vi "SA40144D.20210720 vacuum 1D only.vi"() -> ()   [LabVIEW 2020]
uses:
  <vilib>/Analysis/baseanly.llb/Mean (DBL).vi
  <userlib>/_OpenG.lib/file/file.llb/Build Path - Traditional__ogtk.vi
  <userlib>/LevyLab/LV to ITX/Data/Data.lvclass
  <userlib>/LevyLab/XY Utilities/xy_utilities.lvlib
  <vilib>/Analysis/NI_AALBase.lvlib
panel:
  in  "Tab Control":enum32{"Page 1", "Page 2"}(tab)
  out "G4T vs t  - R Channel":T1(graph)
  out "G2T vs t - R channel":T1(graph)
  out "G2T vs t - X channel":T1(graph)
  out "G4T vs t - X channel":T1(graph)
  out "Temp vs t":T1(graph)
  out "Arrhenius":T1(graph)
  out "R6 - dV":T1(graph)
  out "R5 - I-":T1(graph)
  out "Y6 - dV":T1(graph)
  out "Y5 - I-":T1(graph)
  out "X5 - I-":T1(graph)
  out "X6 - dV":T1(graph)
  in  "Temps to keep (Lifespan)":i32=26
  out "E_a":dbl[](array[numeric])
  in  "Temps to keep (Arrhenius fit)":i32=26
  in  "Source Voltage":dbl=0.1
  in  "Init Temp":i32=275
  in  "Temp Step":i32=5
  in  "Final Temp":i32=400
  in  "Data File":path=path "G:/My Drive/ansom/Data/PPMS 2/SA40144D.20210720/00 - test/SA40144D.20210720.275K.dat"
  in  "Trimming":i32=400
  in  "Update":bool
  in  "OK":bool
  out "error out":errorcluster
  in  "error in (no error)":errorcluster
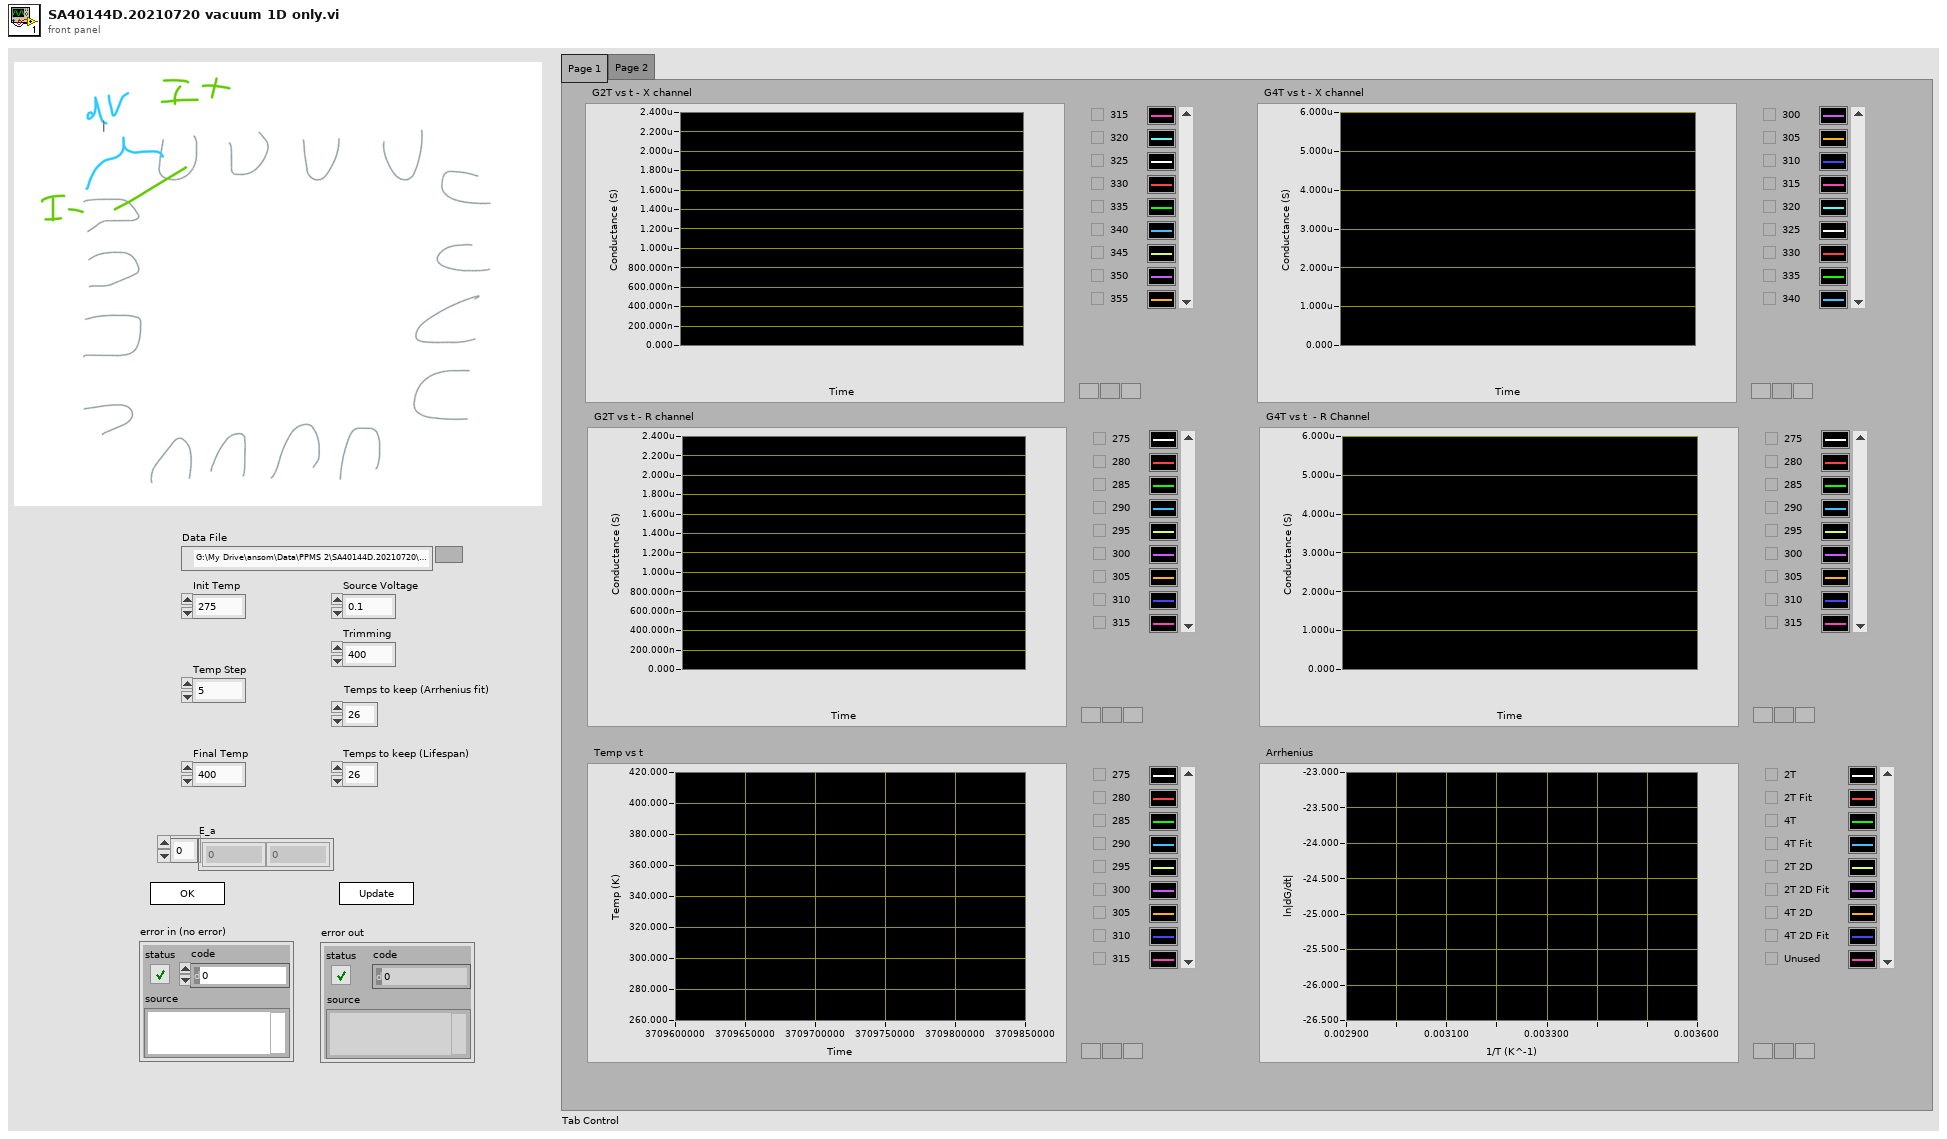
[diagram p1: front panel]
types:
  T1 = cluster{"Data":dbl[], "Best Exponential Fit":dbl[]}[]
  T2 = enum32{"Invalid", "Standard", "Closed", "Hidden", "Minimized", "Maximized"}
  T3 = enum32{"invalid app kind", "Development System", "Run Time System", "Student Edition", "Embedded LabVIEW", "Evaluation", "Custom"}
  T4 = cluster{"Core":cluster{"Current VI Reference":refnum<vi>, "Close Panel on Exit?":bool}, "G2T 1D":cluster{dbl[], dbl[]}[], "G4T 1D":cluster{dbl[], dbl[]}[], "X11":cluster{dbl[], dbl[]}[], "X15":cluster{dbl[], dbl[]}[], "Temp":cluster{dbl[], dbl[]}[], "G2T BG":cluster{dbl[], dbl[]}[], "Source Voltage":dbl, "Final Temp":i32, "Init Temp":i32, "Temp Step":i32, "Data File":path, "Trimming":i32}
  T5 = cluster{"Current VI Reference":refnum<vi>, "Close Panel on Exit?":bool}
  T6 = typedef "Data.lvclass/Dictionary--cluster.ctl" = cluster{"key":string, "value":variant}
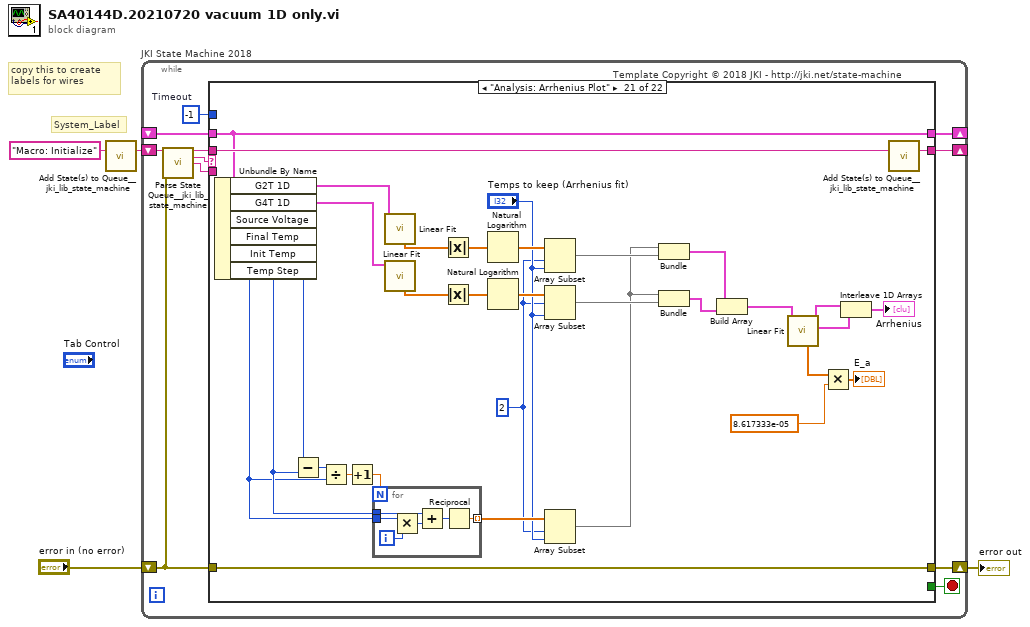
[diagram p0: block diagram]
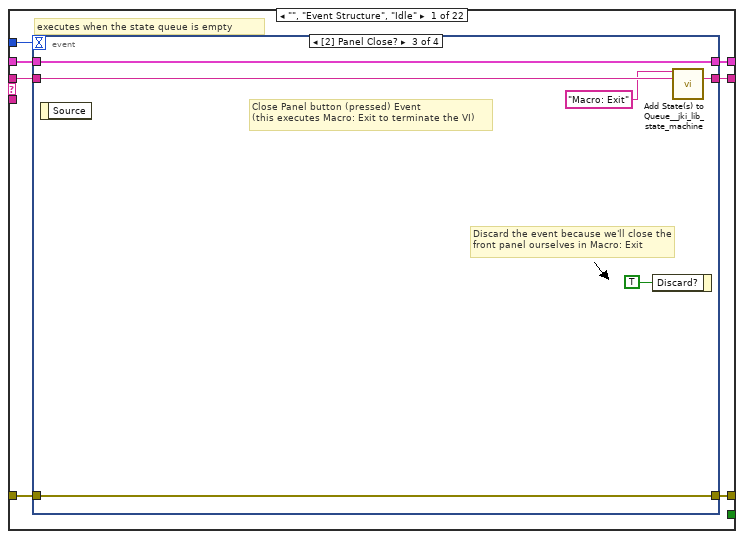
[diagram p2: hidden frame]
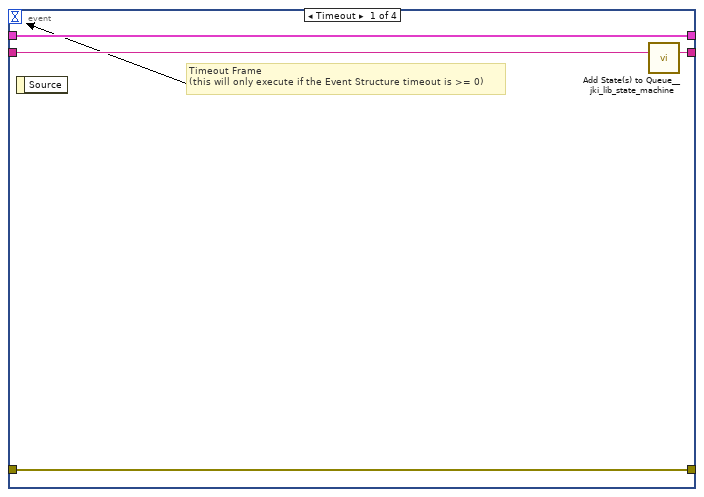
[diagram p3: hidden frame]
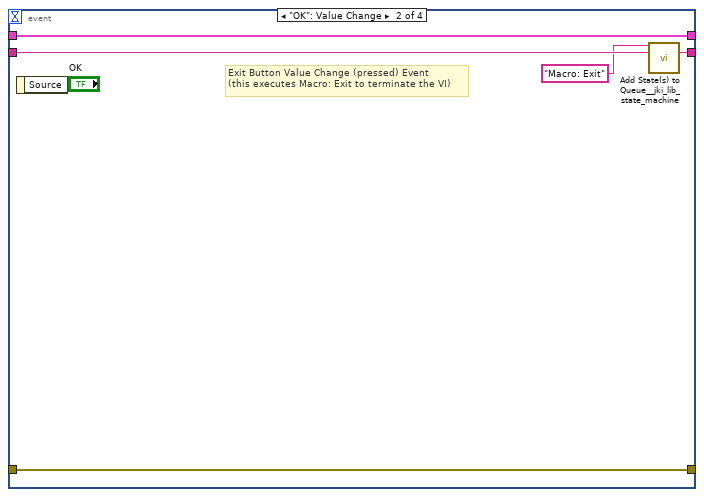
[diagram p4: hidden frame]
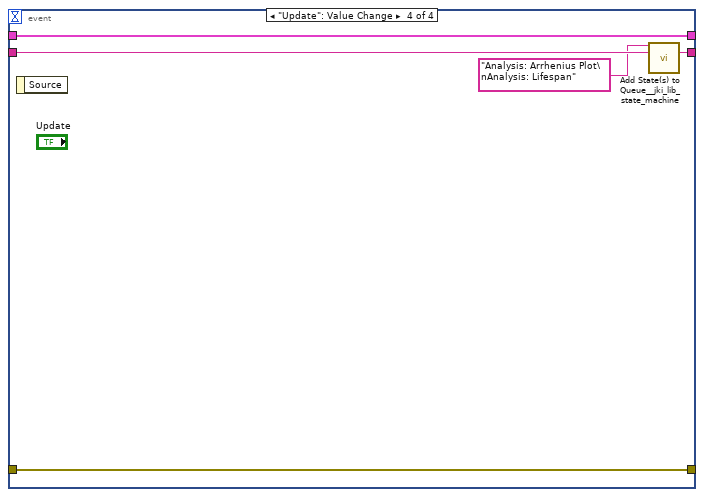
[diagram p5: hidden frame]
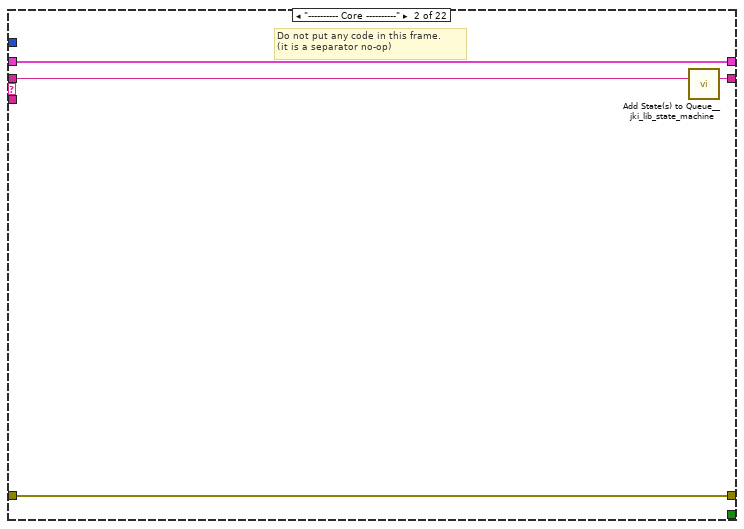
[diagram p6: hidden frame]
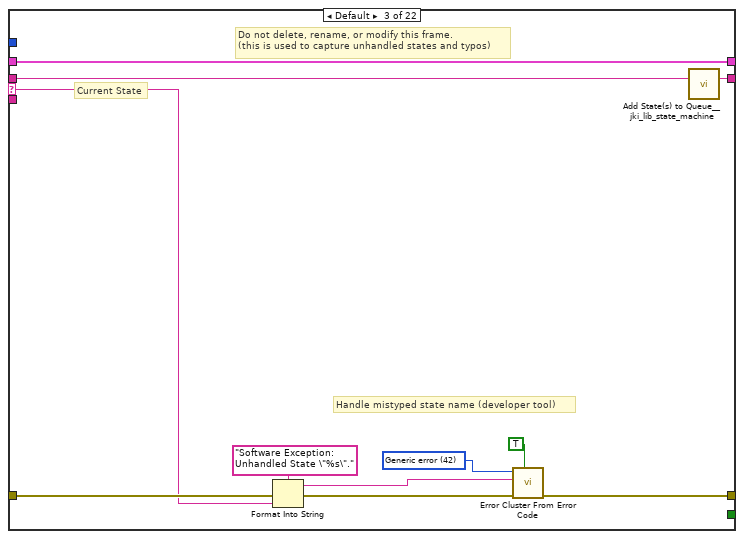
[diagram p7: hidden frame]
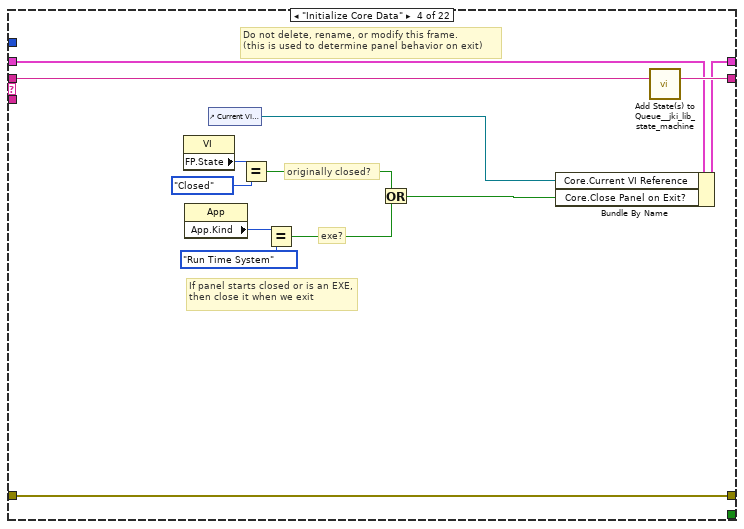
[diagram p8: hidden frame]
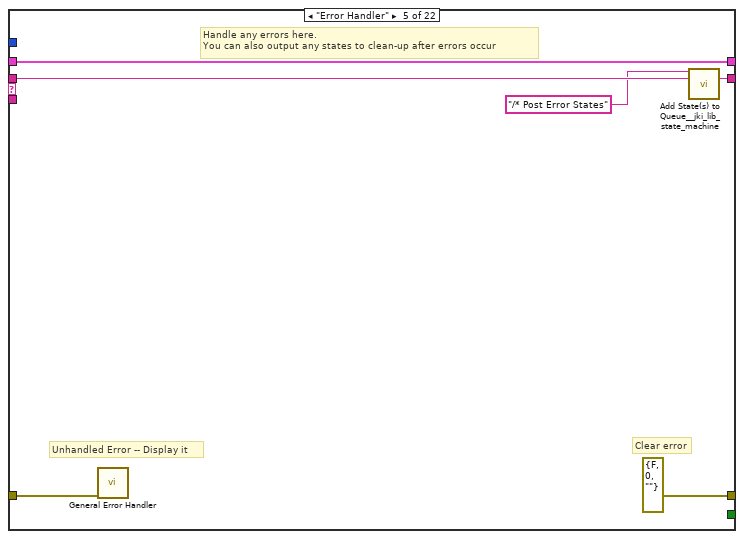
[diagram p9: hidden frame]
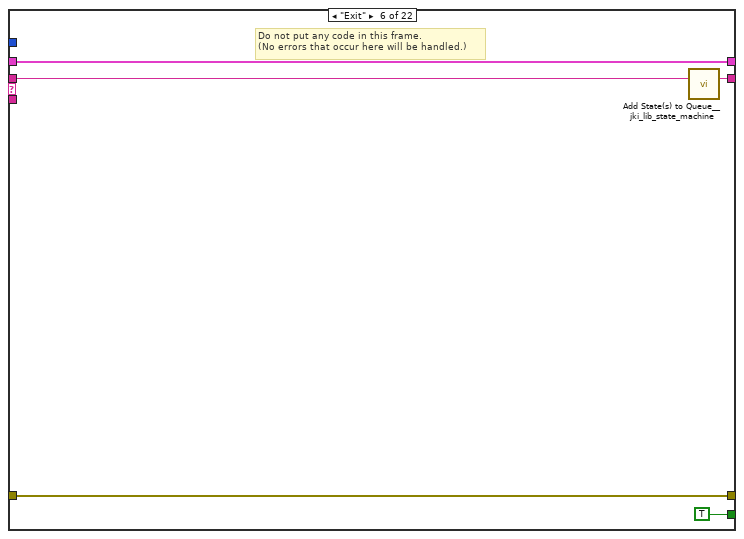
[diagram p10: hidden frame]
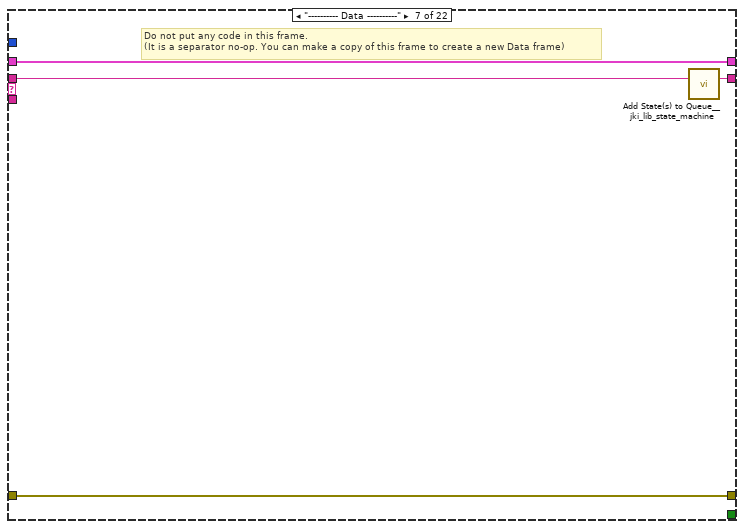
[diagram p11: hidden frame]
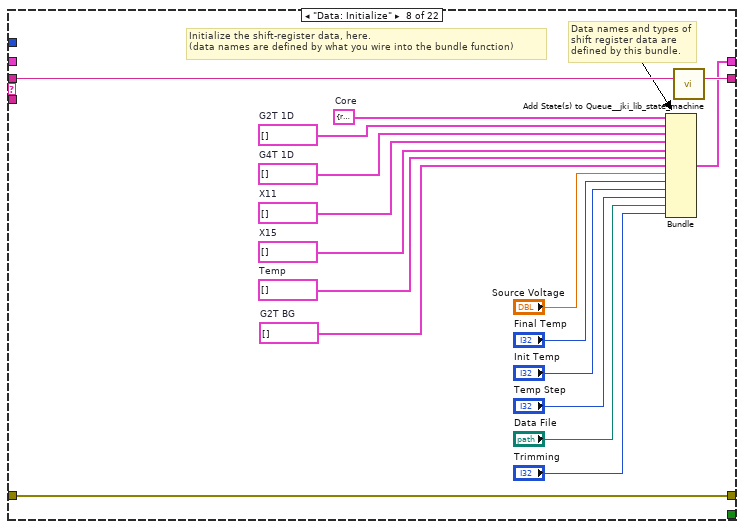
[diagram p12: hidden frame]
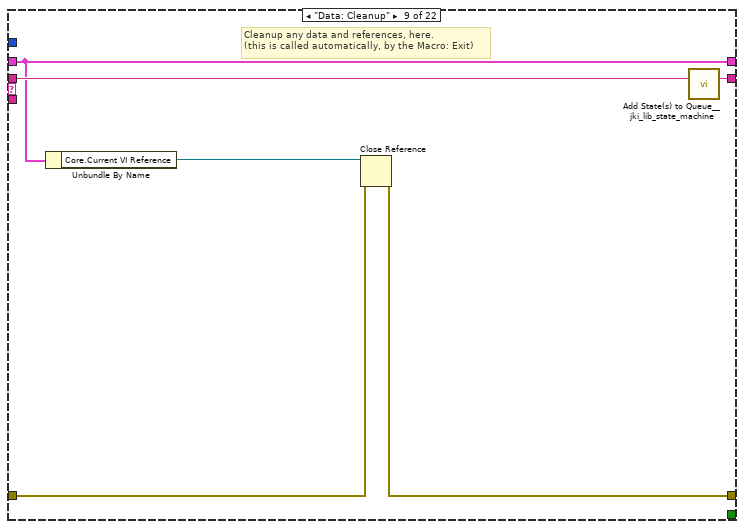
[diagram p13: hidden frame]
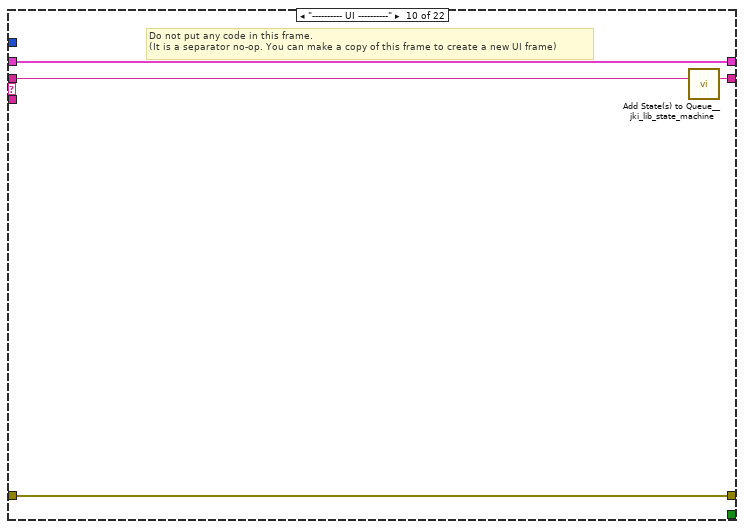
[diagram p14: hidden frame]
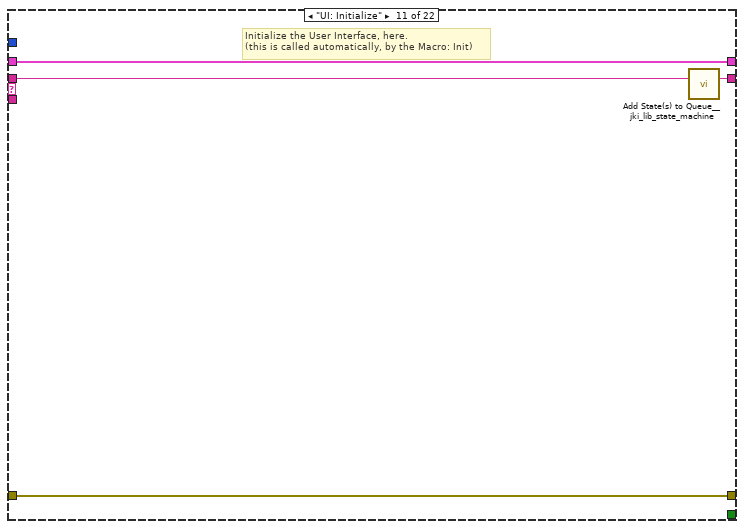
[diagram p15: hidden frame]
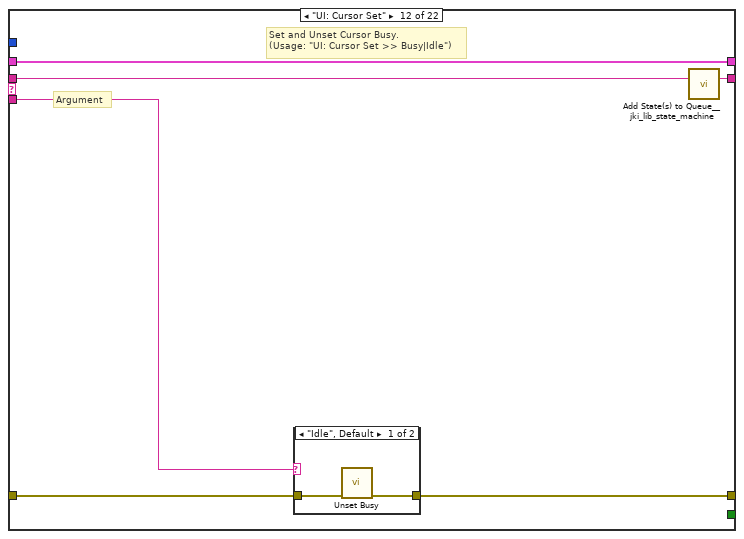
[diagram p16: hidden frame]
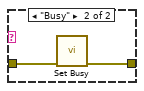
[diagram p17: hidden frame]
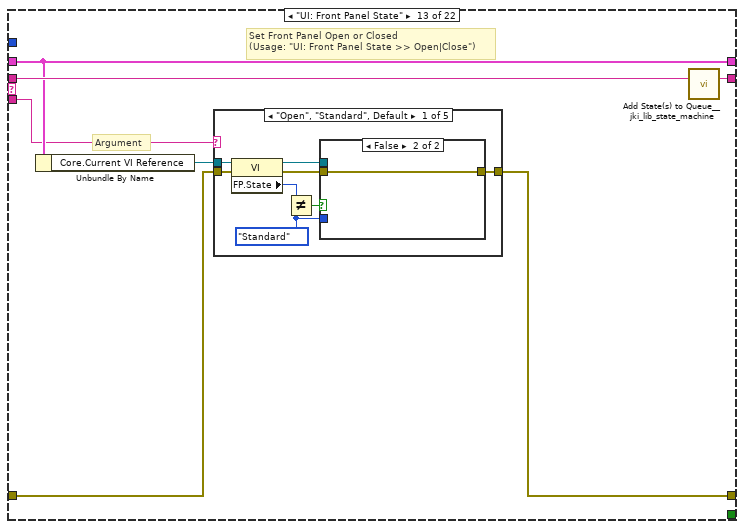
[diagram p18: hidden frame]
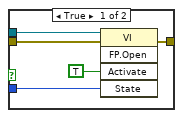
[diagram p19: hidden frame]
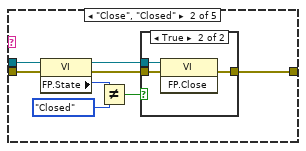
[diagram p20: hidden frame]
diagram:
  # "copy this to create labels for wires"
  # "System_Label"
  n1 = call <vilib>:"Add State(s) to Queue__jki_lib_state_machine.vi"("State(s) in (\"\")"="Macro: Initialize") -> ("States Out"=w4:string)  [unwired: 14 in]
  n2 = while "JKI State Machine 2018" {
    shift-right: [w8] -> _
    shift-left: _ -> [w7]
    shift-right: [w11] -> w1
    shift-left: "error in (no error)" -> [w5]
    shift-right: [w10] -> _
    shift-left: w4 -> [w12]
    stop <- w9 stop-if-true
    w6 = -1  # Timeout
    # "Template Copyright © 2018 JKI - http://jki.net/state-machine"
    n3 = call <vilib>:"Parse State Queue__jki_lib_state_machine.vi"("State Queue"=w12, "Error In (no error)"=w5) -> ("Remaining States"=w14:string, "Current State"=w15:string, "Arguments"=w13:string)  [unwired: 11 in]
    n4 = case shown="\"Analysis: Arrhenius Plot\"" w15 {
      selector: w15 -> [_ _ w47 _ _ _ _ _ _ _ _ _ _ _ _ _ _ _ _ _ _ _]
      tunnel: w14 -> [w22 w46 w51 w70 w76 w81 w85 w102 w108 w112 w116 w122 w133 w202 w207 w217 w221 w242 w315 w359 w392 w430]
      tunnel: w13 -> [_ _ _ _ _ _ _ _ _ _ _ w117 w127 _ _ _ _ _ _ _ _ _]
      tunnel: w7 -> [w20 w43 w49 w63 w73 w79 w82 _ w103 w109 w114 w120 w129 w199 w204 w214 w218 w236 w309 w356 w389 w416]
      tunnel: [w19 w44 w53 w67 errorcluster {"status"=FALSE, "code"=0, "source"=""} ("error out") w78 w83 w99 w104 w110 w113 w118 w130 w200 w205 w215 w219 w238 w311 w357 w390 w428] -> w11
      tunnel: w5 -> [w18 w44 w52 w67 w72 w78 w83 w99 w105 w110 w113 w119 w131 w200 w205 w215 w219 w238 w311 w357 w390 w428]
      tunnel: [w21 w45 w50 w69 w75 w80 w84 w101 w107 w111 w115 w121 w132 w201 w206 w216 w220 w241 w314 w358 w391 w429] -> w10
      tunnel: [_ _ _ _ _ TRUE _ _ _ _ _ _ _ _ _ _ _ _ _ _ _ _] -> w9
      tunnel: [w17 w43 w49 w68 w73 w79 w82 w100 w103 w109 w114 w120 w129 w199 w204 w214 w218 w237 w310 w356 w389 w416] -> w8
      tunnel: w6 -> [w16 _ _ _ _ _ _ _ _ _ _ _ _ _ _ _ _ _ _ _ _ _]
      frame "", "Event Structure", "Idle" {
        # "executes when the state queue is empty"
        n5 = event shown="[2] Panel Close?" {
          selector: _ -> [_ _ _ _]
          dyn-events: _ -> [_ _ _ _]
          timeout: w16 -> [_ _ _ _]
          tunnel: w22 -> [w26 w31 w37 w41]
          tunnel: [w25 w30 w36 w40] -> w21
          tunnel: w20 -> [w23 w28 w34 w42]
          tunnel: [w24 w29 w35 w38] -> w19
          tunnel: w18 -> [w24 w29 w35 w38]
          tunnel: [w23 w28 w34 w42] -> w17
          event Timeout {
            # "Timeout Frame\n(this will only execute if the Event Structure timeout is >= 0)"
            n6 = event-data() -> ()  [unwired: 1 in, 1 out]
            n7 = call <vilib>:"Add State(s) to Queue__jki_lib_state_machine.vi"("State(s) in (\"\")"=w26) -> ("States Out"=w25:string)  [unwired: 14 in]
          }
          event "OK": Value Change {
            # "Exit Button Value Change (pressed) Event\n(this executes Macro: Exit to terminate the VI)"
            n8 = event-data() -> ()  [unwired: 1 in, 1 out]
            n9 = call <vilib>:"Add State(s) to Queue__jki_lib_state_machine.vi"("State(s) in Front (\"\")"="Macro: Exit", "State(s) in (\"\")"=w31) -> ("States Out"=w30:string)  [unwired: 13 in]
          }
          event Panel Close? {
            # "Discard the event because we'll close the front panel ourselves in Macro: Exit"
            # "Close Panel button (pressed) Event\n(this executes Macro: Exit to terminate the VI)"
            n10 = event-data() -> ()  [unwired: 1 in, 1 out]
            n11 = event-data("Discard?"=TRUE) -> ()  [unwired: 1 in, 1 out]
            n12 = call <vilib>:"Add State(s) to Queue__jki_lib_state_machine.vi"("State(s) in Front (\"\")"="Macro: Exit", "State(s) in (\"\")"=w37) -> ("States Out"=w36:string)  [unwired: 13 in]
          }
          event "Update": Value Change {
            n13 = event-data() -> ()  [unwired: 1 in, 1 out]
            n14 = call <vilib>:"Add State(s) to Queue__jki_lib_state_machine.vi"("State(s) in Front (\"\")"="Analysis: Arrhenius Plot\nAnalysis: Lifespan" ("State(s) in Front (\"\")"), "State(s) in (\"\")"=w41) -> ("States Out"=w40:string)  [unwired: 13 in]
          }
        }
      }
      frame "---------- Core ----------" {
        # "Do not put any code in this frame.\n(it is a separator no-op)"
        n15 = call <vilib>:"Add State(s) to Queue__jki_lib_state_machine.vi"("State(s) in (\"\")"=w46) -> ("States Out"=w45:string)  [unwired: 14 in]
      }
      frame Default {
        w56 = 42 items=["No error", "Argument error", "Memory is full", "Out of zone", "End of file", "File already open", "Generic file I/O error", "File not found", "File permission error", "Disk is full", "Duplicate path", "Too many files open", "System feature not enabled", "Resource file not found", "Cannot add resource", "Resource not found", "Image not found", "Image memory error", "Pen does not exist", "Config type invalid", "Config token not found", "Config parse error", "Config memory error", "Bad external code format", "Bad external code offset", "External code not present", "Null window", "Destroy window error", "Null menu", "Print aborted", "Bad print record", "Print driver error", "Windows error during printing", "Memory error during printing", "Print dialog error", "Generic print error", "Invalid device refnum", "Device not found", "Device parameter error", "Device unit error", "Cannot open device", "Device call aborted", "Generic error", "Cancelled by user", "Object ID too low", "Object ID too high", "Object not in heap", "Unknown heap", "Unknown object (invalid DefProc)", "Unknown object (DefProc not in table)", "Message out of range", "Invalid (null) method", "Unknown message", "Manager call not supported", "Bad address", "Network operation in progress", "Network operation timed out", "Connection is busy", "Network attribute not supported", "Network error", "Address in use", "System out of memory", "Connection aborted", "Connection refused", "Not connected", "Already connected", "Connection closed", "Initialization error (interapplication manager)", "Bad occurrence", "Wait on unbound occurrence handler", "Occurrence queue overflow", "Datalog type conflict", "Unused", "Unrecognized type (interapplication manager)", "Memory corrupt", "Failed to make temporary DLL", "Old CIN version", "Drag socket not found", "Failed to load drop-object", "Failed to register OLE object", "Failed to release OLE object", "Format specifier type mismatch", "Unknown format specifier", "Too few format specifiers", "Too many format specifiers", "Scan failed", "Newer CIN version", "Error converting to variant", "Runtime menu error", "Password tampered", "Variant attribute not found", "Incompatible variant data type", "Event data is not available", "Event Store is not present", "Occurrence is not found", "Event Queue is not created", "Event info is not available", "Refnum passed is NULL", "Error retrieving Class GUID", "Error retrieving CoClass GUID", "Error retrieving TypeLib GUID.", "Bad built application magic bytes.", "Specific driver is different from the specific driver associated with the Logical Name.", "There is no session opened to the class driver.", "Max Error", "MAX - Error with config objects", "MAX - Error loading configuration", "MAX - Group not supported"]
        # "Current State"
        # "Do not delete, rename, or modify this frame.\n(this is used to capture unhandled states and typos)"
        # "Handle mistyped state name (developer tool)"
        n16 = Format Into String(format string="Software Exception: Unhandled State \"%s\"." ("message"), error in=w52, w47) -> (resulting string=w55:string, error out=w54:errorcluster)  [unwired: 1 in]
        n17 = call <vilib>:"Error Cluster From Error Code.vi"("show call chain? (False)"=TRUE, "error in (no error)"=w54, "error message (\"\")"=w55, "error code (0)"=w56) -> ("error out"=w53:errorcluster)  [unwired: 5 in]
        n18 = call <vilib>:"Add State(s) to Queue__jki_lib_state_machine.vi"("State(s) in (\"\")"=w51) -> ("States Out"=w50:string)  [unwired: 14 in]
      }
      frame "Initialize Core Data" {
        # "Do not delete, rename, or modify this frame.\n(this is used to determine panel behavior on exit)"
        # "originally closed?"
        # "exe?"
        # "If panel starts closed or is an EXE, then close it when we exit"
        n19 = property class="VI"() -> ("FP.State"=w60:T2)  [unwired: 2 in, 2 out]
        n20 = property class="App"() -> ("App.Kind"=w66:T3)  [unwired: 2 in, 2 out]
        n21 = control-ref of="Current VI Reference"() -> (w61:refnum<vi>)
        n22 = Equal?(x=w60, y=T2."Closed" ("Front Panel Window:State")) -> (x = y?=w58:bool)
        n23 = Equal?(x=w66, y=T3."Run Time System" ("Application:Kind")) -> (x = y?=w64:bool)
        n24 = Or(x=w58, y=w64) -> (x .or. y?=w62:bool)
        n25 = Bundle By Name(cluster=w63, "Core.Current VI Reference"=w61, "Core.Close Panel on Exit?"=w62) -> (w68:T4)
        n26 = call <vilib>:"Add State(s) to Queue__jki_lib_state_machine.vi"("State(s) in (\"\")"=w70) -> ("States Out"=w69:string)  [unwired: 14 in]
      }
      frame "Error Handler" {
        # "Unhandled Error -- Display it"
        # "Handle any errors here.\nYou can also output any states to clean-up after errors occur"
        # "Clear error"
        n27 = call <vilib>:"General Error Handler.vi"("error in (no error)"=w72) -> ()  [unwired: 10 in, 5 out]
        n28 = call <vilib>:"Add State(s) to Queue__jki_lib_state_machine.vi"("State(s) in Front (\"\")"="/* Post Error States", "State(s) in (\"\")"=w76) -> ("States Out"=w75:string)  [unwired: 13 in]
      }
      frame "Exit" {
        # "Do not put any code in this frame.\n(No errors that occur here will be handled.)"
        n29 = call <vilib>:"Add State(s) to Queue__jki_lib_state_machine.vi"("State(s) in (\"\")"=w81) -> ("States Out"=w80:string)  [unwired: 14 in]
      }
      frame "---------- Data ----------" {
        # "Do not put any code in this frame.\n(It is a separator no-op. You can make a copy of this frame to create a new Data frame)"
        n30 = call <vilib>:"Add State(s) to Queue__jki_lib_state_machine.vi"("State(s) in (\"\")"=w85) -> ("States Out"=w84:string)  [unwired: 14 in]
      }
      frame "Data: Initialize" {
        w86 = cluster{dbl[], dbl[]}[] []  # G2T BG
        w87 = cluster{dbl[], dbl[]}[] []  # Temp
        w96 = cluster{dbl[], dbl[]}[] []  # X15
        w95 = cluster{dbl[], dbl[]}[] []  # X11
        w94 = cluster{dbl[], dbl[]}[] []  # G4T 1D
        w93 = cluster{dbl[], dbl[]}[] []  # G2T 1D
        w98 = T5 {"Current VI Reference"=refnum, "Close Panel on Exit?"=FALSE}  # Core
        # "Data names and types of shift register data are defined by this bundle."
        # "Initialize the shift-register data, here.\n(data names are defined by what you wire into the bundle function)"
        n31 = Bundle("Core"=w98, "G2T 1D"=w93, "G4T 1D"=w94, "X11"=w95, "X15"=w96, "Temp"=w87, "G2T BG"=w86, "Source Voltage"="Source Voltage", "Final Temp"="Final Temp", "Init Temp"="Init Temp", "Temp Step"="Temp Step", "Data File"="Data File", "Trimming"="Trimming") -> (w100:T4)  [unwired: 1 in]
        n32 = call <vilib>:"Add State(s) to Queue__jki_lib_state_machine.vi"("State(s) in (\"\")"=w102) -> ("States Out"=w101:string)  [unwired: 14 in]
      }
      frame "Data: Cleanup" {
        # "Cleanup any data and references, here.\n(this is called automatically, by the Macro: Exit)"
        n33 = Unbundle By Name(w103) -> ("Core.Current VI Reference"=w106:refnum<vi>)
        n34 = Close Reference(reference=w106, error in (no error)=w105) -> (error out=w104:errorcluster)
        n35 = call <vilib>:"Add State(s) to Queue__jki_lib_state_machine.vi"("State(s) in (\"\")"=w108) -> ("States Out"=w107:string)  [unwired: 14 in]
      }
      frame "---------- UI ----------" {
        # "Do not put any code in this frame.\n(It is a separator no-op. You can make a copy of this frame to create a new UI frame)"
        n36 = call <vilib>:"Add State(s) to Queue__jki_lib_state_machine.vi"("State(s) in (\"\")"=w112) -> ("States Out"=w111:string)  [unwired: 14 in]
      }
      frame "UI: Initialize" {
        # "Initialize the User Interface, here.\n(this is called automatically, by the Macro: Init)"
        n37 = call <vilib>:"Add State(s) to Queue__jki_lib_state_machine.vi"("State(s) in (\"\")"=w116) -> ("States Out"=w115:string)  [unwired: 14 in]
      }
      frame "UI: Cursor Set" {
        # "Argument"
        # "Set and Unset Cursor Busy.\n(Usage: \"UI: Cursor Set >> Busy|Idle\")"
        n38 = case shown="\"Idle\", Default" w117 {
          tunnel: w119 -> [w124 w126]
          tunnel: [w123 w125] -> w118
          frame "Idle", Default {
            n39 = call <vilib>:"Unset Busy.vi"("error in (no error)"=w124) -> ("error out"=w123:errorcluster)  [unwired: 10 in]
          }
          frame "Busy" {
            n40 = call <vilib>:"Set Busy.vi"("error in (no error)"=w126) -> ("error out"=w125:errorcluster)  [unwired: 9 in, 1 out]
          }
        }
        n41 = call <vilib>:"Add State(s) to Queue__jki_lib_state_machine.vi"("State(s) in (\"\")"=w122) -> ("States Out"=w121:string)  [unwired: 14 in]
      }
      frame "UI: Front Panel State" {
        # "Argument"
        # "Set Front Panel Open or Closed\n(Usage: \"UI: Front Panel State >> Open|Close\")"
        n42 = Unbundle By Name(w129) -> ("Core.Current VI Reference"=w128:refnum<vi>)
        n43 = case shown="\"Open\", \"Standard\", Default" w127 {
          tunnel: w131 -> [w139 w154 w165 w178 w191]
          tunnel: [w141 w155 w167 w180 w193] -> w130
          tunnel: w128 -> [w140 w152 w166 w179 w192]
          frame "Open", "Standard", Default {
            w134 = T2."Standard" ("State")
            n44 = property class="VI"(reference=w140, error in=w139) -> (reference out=w137:refnum<vi>, error out=w138:errorcluster, "FP.State"=w136:T2)
            n45 = Not Equal?(x=w136, y=w134) -> (x != y?=w135:bool)
            n46 = case shown="False" w135 {
              tunnel: [w145 w147] -> w141
              tunnel: w138 -> [w144 w147]
              tunnel: w137 -> [w143 _]
              tunnel: w134 -> [w142 _]
              frame True {
                n47 = invoke class="VI" method="FP.Open"(reference=w143, error in=w144, "Activate"=TRUE, "State"=w142) -> (error out=w145:errorcluster)  [unwired: 1 in, 4 out]
              }
              frame False {
              }
            }
          }
          frame "Close", "Closed" {
            n48 = property class="VI"(reference=w152, error in=w154) -> (reference out=w151:refnum<vi>, error out=w153:errorcluster, "FP.State"=w149:T2)
            n49 = Not Equal?(x=w149, y=T2."Closed" ("Front Panel Window:State")) -> (x != y?=w148:bool)
            n50 = case shown="True" w148 {
              tunnel: [w156 w159] -> w155
              tunnel: w153 -> [w156 w158]
              tunnel: w151 -> [_ w157]
              frame False {
              }
              frame True {
                n51 = invoke class="VI" method="FP.Close"(reference=w157, error in=w158) -> (error out=w159:errorcluster)  [unwired: 1 in, 2 out]
              }
            }
          }
          frame "Hidden", "Hide" {
            w160 = T2."Hidden" ("State")
            n52 = property class="VI"(reference=w166, error in=w165) -> (reference out=w163:refnum<vi>, error out=w164:errorcluster, "FP.State"=w162:T2)
            n53 = Not Equal?(x=w162, y=w160) -> (x != y?=w161:bool)
            n54 = case shown="True" w161 {
              tunnel: [w171 w172] -> w167
              tunnel: w164 -> [w170 w172]
              tunnel: w163 -> [w169 _]
              tunnel: w160 -> [w168 _]
              frame True {
                n55 = invoke class="VI" method="FP.Open"(reference=w169, error in=w170, "State"=w168) -> (error out=w171:errorcluster)  [unwired: 2 in, 4 out]
              }
              frame False {
              }
            }
          }
          frame "Minimize", "Minimized" {
            w173 = T2."Minimized" ("State")
            n56 = property class="VI"(reference=w179, error in=w178) -> (reference out=w176:refnum<vi>, error out=w177:errorcluster, "FP.State"=w175:T2)
            n57 = Not Equal?(x=w175, y=w173) -> (x != y?=w174:bool)
            n58 = case shown="True" w174 {
              tunnel: [w184 w185] -> w180
              tunnel: w177 -> [w183 w185]
              tunnel: w176 -> [w182 _]
              tunnel: w173 -> [w181 _]
              frame True {
                n59 = invoke class="VI" method="FP.Open"(reference=w182, error in=w183, "State"=w181) -> (error out=w184:errorcluster)  [unwired: 2 in, 4 out]
              }
              frame False {
              }
            }
          }
          frame "Maximize", "Maximized" {
            w186 = T2."Maximized" ("State")
            n60 = property class="VI"(reference=w192, error in=w191) -> (reference out=w189:refnum<vi>, error out=w190:errorcluster, "FP.State"=w188:T2)
            n61 = Not Equal?(x=w188, y=w186) -> (x != y?=w187:bool)
            n62 = case shown="True" w187 {
              tunnel: [w197 w198] -> w193
              tunnel: w190 -> [w196 w198]
              tunnel: w189 -> [w195 _]
              tunnel: w186 -> [w194 _]
              frame True {
                n63 = invoke class="VI" method="FP.Open"(reference=w195, error in=w196, "State"=w194) -> (error out=w197:errorcluster)  [unwired: 2 in, 4 out]
              }
              frame False {
              }
            }
          }
        }
        n64 = call <vilib>:"Add State(s) to Queue__jki_lib_state_machine.vi"("State(s) in (\"\")"=w133) -> ("States Out"=w132:string)  [unwired: 14 in]
      }
      frame "---------- Macro ----------" {
        # "Do not put any code in this frame.\n(It is a separator no-op. You can make a copy of this frame to create a new Macro frame)"
        n65 = call <vilib>:"Add State(s) to Queue__jki_lib_state_machine.vi"("State(s) in (\"\")"=w202) -> ("States Out"=w201:string)  [unwired: 14 in]
      }
      frame "Macro: Initialize" {
        # "Initialization Macro\n(This is called once, when the VI starts)"
        n66 = call <vilib>:"Add State(s) to Queue__jki_lib_state_machine.vi"("State(s) in Front (\"\")"="Data: Initialize\nInitialize Core Data\nUI: Initialize\nUI: Front Panel State >> Open\nAnalysis: Load 1D\nAnalysis: Load X\nAnalysis: Plot G vs t\nAnalysis: Arrhenius Plot\nAnalysis: Lifespan", "State(s) in (\"\")"=w207) -> ("States Out"=w206:string)  [unwired: 13 in]
      }
      frame "Macro: Exit" {
        # "Exit Macro\n(This is called once, when the VI exits)"
        n67 = Unbundle By Name(w214) -> ("Core.Close Panel on Exit?"=w213:bool)
        n68 = Select(t="UI: Front Panel State >> Close", s=w213, f="") -> (s? t:f=w210:string)
        n69 = call <vilib>:"Add State(s) to Queue__jki_lib_state_machine.vi"("State(s) in (\"\")"=w210, "State(s) at Back (\"\")"="Data: Cleanup\nExit") -> ("States Out"=w208:string)  [unwired: 13 in]
        n70 = call <vilib>:"Add State(s) to Queue__jki_lib_state_machine.vi"("State(s) in Front (\"\")"=w208, "State(s) in (\"\")"=w217) -> ("States Out"=w216:string)  [unwired: 13 in]
      }
      frame "---------- Analysis ----------" {
        # "Template Separator\n(You can make a copy of, or modify, this frame)"
        n71 = call <vilib>:"Add State(s) to Queue__jki_lib_state_machine.vi"("State(s) in (\"\")"=w221) -> ("States Out"=w220:string)  [unwired: 14 in]
      }
      frame "Analysis: Load 1D" {
        n72 = Unbundle By Name(w236) -> ("Source Voltage"=w235:dbl, "Final Temp"=w232:i32, "Init Temp"=w229:i32, "Temp Step"=w228:i32, "Data File"=w230:path, "Trimming"=w227:i32)
        n73 = Subtract(x=w232, y=w229) -> (x-y=w239:i32)
        n74 = Divide(x=w239, y=w228) -> (x/y=w240:dbl)
        n75 = Increment(x=w240) -> (x+1=w231:dbl)
        n76 = for {
          N: w231 -> [_]
          tunnel: w235 -> [w250]
          tunnel: [w286] -> w234 mode=indexing
          tunnel: [w285] -> w233 mode=indexing
          tunnel: w230 -> [w284]
          tunnel: w229 -> [w283]
          tunnel: w228 -> [w282]
          tunnel: w227 -> [w263]
          tunnel: [w280] -> w226 mode=indexing
          tunnel: [w252] -> w225 mode=indexing
          tunnel: [w251] -> w224 mode=indexing
          tunnel: [w244] -> w223 mode=indexing
          tunnel: [w243] -> w222 mode=indexing
          i -> [w289]
          n77 = Strip Path(path=w284) -> (stripped path=w294:path, name=w293:string)
          n78 = Multiply(x=w282, y=w289) -> (x*y=w290:i32)
          n79 = Add(x=w283, y=w290) -> (x+y=w295:i32)
          n80 = String Subset(string=w293, length (rest)=18) -> (substring=w291:string)  [unwired: 1 in]
          n81 = Format Into String(w295) -> (resulting string=w297:string)  [unwired: 3 in, 1 out]
          n82 = Concatenate Strings(w291, w297, "K.dat" ("string")) -> (w296:string)
          n83 = call-poly <userlib>:"Build Path__ogtk.vi"("name or relative path"=w296, "base path"=w294) -> ("appended path"=w298:path)
          n84 = call <userlib>:"Data Read.vi"("path"=w298) -> ("Data (Dictionary)"=w266:T6[])  [unwired: 7 in, 3 out]
          n85 = call "Read Dictionary.vi"("Numeric"=0, "Dictionary In"=w266) -> ("data"=w276:dbl[])
          n86 = call "Read Dictionary.vi"("Numeric"=7 ("index"), "Dictionary In"=w266) -> ("data"=w272:dbl[])
          n87 = call "Read Dictionary.vi"("Numeric"=15 ("index"), "Dictionary In"=w266) -> ("data"=w265:dbl[])
          n88 = call "Read Dictionary.vi"("Numeric"=8, "Dictionary In"=w266) -> ("data"=w275:dbl[])
          n89 = call "Read Dictionary.vi"("Numeric"=16 ("index"), "Dictionary In"=w266) -> ("data"=w264:dbl[])
          n90 = call "Read Dictionary.vi"("Numeric"=1, "Dictionary In"=w266) -> ("data"=w274:dbl[])
          n91 = Array Subset(array=w276, index=w263) -> (w247:dbl[])  [unwired: 1 in]
          n92 = Array Subset(array=w272, index=w263) -> (w262:dbl[])  [unwired: 1 in]
          n93 = Array Subset(array=w265, index=w263) -> (w261:dbl[])  [unwired: 1 in]
          n94 = Array Subset(array=w275, index=w263) -> (w260:dbl[])  [unwired: 1 in]
          n95 = Array Subset(array=w264, index=w263) -> (w259:dbl[])  [unwired: 1 in]
          n96 = Square(x=w262) -> (x^2=w258:dbl[])
          n97 = Square(x=w261) -> (x^2=w257:dbl[])
          n98 = Square(x=w260) -> (x^2=w255:dbl[])
          n99 = Square(x=w259) -> (x^2=w254:dbl[])
          n100 = Add(x=w258, y=w257) -> (x+y=w256:dbl[])
          n101 = Add(x=w255, y=w254) -> (x+y=w253:dbl[])
          n102 = Square Root(x=w256) -> (sqrt(x)=w249:dbl[])
          n103 = Square Root(x=w253) -> (sqrt(x)=w248:dbl[])
          n104 = Bundle(w247, w249) -> (w252:cluster{dbl[], dbl[]})  [unwired: 1 in]
          n105 = Bundle(w247, w248) -> (w251:cluster{dbl[], dbl[]})  [unwired: 1 in]
          n106 = Divide(x=w262, y=w250) -> (x/y=w288:dbl[])
          n107 = Divide(x=w249, y=w250) -> (x/y=w245:dbl[])
          n108 = Array Subset(array=w274) -> (w281:dbl[])  [unwired: 2 in]
          n109 = Absolute Value(x=w288) -> (abs(x)=w271:dbl[])
          n110 = Divide(x=w249, y=w248) -> (x/y=w246:dbl[])
          n111 = Divide(x=w262, y=w260) -> (x/y=w269:dbl[])
          n112 = Bundle(w247, w245) -> (w244:cluster{dbl[], dbl[]})  [unwired: 1 in]
          n113 = Bundle(w247, w271) -> (w286:cluster{dbl[], dbl[]})  [unwired: 1 in]
          n114 = Bundle(w247, w281) -> (w280:cluster{dbl[], dbl[]})  [unwired: 1 in]
          n115 = Absolute Value(x=w269) -> (abs(x)=w270:dbl[])
          n116 = Bundle(w247, w246) -> (w243:cluster{dbl[], dbl[]})  [unwired: 1 in]
          n117 = Bundle(w247, w270) -> (w285:cluster{dbl[], dbl[]})  [unwired: 1 in]
        }
        "R5 - I-" <- w225
        "R6 - dV" <- w224
        "G2T vs t - R channel" <- w223
        "G4T vs t  - R Channel" <- w222
        n118 = call <vilib>:"Add State(s) to Queue__jki_lib_state_machine.vi"("State(s) in (\"\")"=w242) -> ("States Out"=w241:string)  [unwired: 14 in]
        n119 = Bundle By Name(cluster=w236, "G2T 1D"=w234, "G4T 1D"=w233, "Temp"=w226) -> (w237:T4)
      }
      frame "Analysis: Load X" {
        n120 = Unbundle By Name(w309) -> ("Final Temp"=w307:i32, "Init Temp"=w304:i32, "Temp Step"=w303:i32, "Data File"=w305:path, "Trimming"=w302:i32)  [unwired: 1 out]
        n121 = Subtract(x=w307, y=w304) -> (x-y=w312:i32)
        n122 = Divide(x=w312, y=w303) -> (x/y=w313:dbl)
        n123 = Increment(x=w313) -> (x+1=w306:dbl)
        n124 = for {
          N: w306 -> [_]
          tunnel: [w339] -> w301 mode=indexing
          tunnel: [w338] -> w308 mode=indexing
          tunnel: w305 -> [w337]
          tunnel: w304 -> [w336]
          tunnel: w303 -> [w335]
          tunnel: w302 -> [w321]
          tunnel: [w317] -> w300 mode=indexing
          tunnel: [w316] -> w299 mode=indexing
          i -> [w341]
          n125 = Strip Path(path=w337) -> (stripped path=w346:path, name=w345:string)
          n126 = Multiply(x=w335, y=w341) -> (x*y=w342:i32)
          n127 = Add(x=w336, y=w342) -> (x+y=w347:i32)
          n128 = String Subset(string=w345, length (rest)=18) -> (substring=w343:string)  [unwired: 1 in]
          n129 = Format Into String(w347) -> (resulting string=w349:string)  [unwired: 3 in, 1 out]
          n130 = Concatenate Strings(w343, w349, "K.dat" ("string")) -> (w348:string)
          n131 = call-poly <userlib>:"Build Path__ogtk.vi"("name or relative path"=w348, "base path"=w346) -> ("appended path"=w350:path)
          n132 = call <userlib>:"Data Read.vi"("path"=w350) -> ("Data (Dictionary)"=w326:T6[])  [unwired: 7 in, 3 out]
          n133 = call "Read Dictionary.vi"("Numeric"=0, "Dictionary In"=w326) -> ("data"=w332:dbl[])
          n134 = call "Read Dictionary.vi"("Numeric"=7 ("index"), "Dictionary In"=w326) -> ("data"=w329:dbl[])
          n135 = call "Read Dictionary.vi"("Numeric"=8, "Dictionary In"=w326) -> ("data"=w331:dbl[])
          n136 = call "Read Dictionary.vi"("Numeric"=15, "Dictionary In"=w326) -> ("data"=w323:dbl[])
          n137 = call "Read Dictionary.vi"("Numeric"=16, "Dictionary In"=w326) -> ("data"=w322:dbl[])
          n138 = Array Subset(array=w332, index=w321) -> (w318:dbl[])  [unwired: 1 in]
          n139 = Array Subset(array=w329, index=w321) -> (w327:dbl[])  [unwired: 1 in]
          n140 = Array Subset(array=w331, index=w321) -> (w328:dbl[])  [unwired: 1 in]
          n141 = Array Subset(array=w323, index=w321) -> (w320:dbl[])  [unwired: 1 in]
          n142 = Array Subset(array=w322, index=w321) -> (w319:dbl[])  [unwired: 1 in]
          n143 = Bundle(w318, w320) -> (w317:cluster{dbl[], dbl[]})  [unwired: 1 in]
          n144 = Bundle(w318, w319) -> (w316:cluster{dbl[], dbl[]})  [unwired: 1 in]
          n145 = Bundle(w318, w327) -> (w339:cluster{dbl[], dbl[]})  [unwired: 1 in]
          n146 = Bundle(w318, w328) -> (w338:cluster{dbl[], dbl[]})  [unwired: 1 in]
        }
        "Y6 - dV" <- w299
        "Y5 - I-" <- w300
        n147 = call <vilib>:"Add State(s) to Queue__jki_lib_state_machine.vi"("State(s) in (\"\")"=w315) -> ("States Out"=w314:string)  [unwired: 14 in]
        n148 = Bundle By Name(cluster=w309, "X11"=w301, "X15"=w308) -> (w310:T4)
      }
      frame "Analysis: Plot G vs t" {
        n149 = Unbundle By Name(w356) -> ("G2T 1D"=→"G2T vs t - X channel":cluster{dbl[], dbl[]}[], "G4T 1D"=→"G4T vs t - X channel":cluster{dbl[], dbl[]}[], "X11"=→"X5 - I-":cluster{dbl[], dbl[]}[], "X15"=→"X6 - dV":cluster{dbl[], dbl[]}[], "Temp"=→"Temp vs t":cluster{dbl[], dbl[]}[])
        n150 = call <vilib>:"Add State(s) to Queue__jki_lib_state_machine.vi"("State(s) in (\"\")"=w359) -> ("States Out"=w358:string)  [unwired: 14 in]
      }
      frame "Analysis: Arrhenius Plot" {
        w360 = 2
        n151 = Unbundle By Name(w389) -> ("G2T 1D"=w364:cluster{dbl[], dbl[]}[], "G4T 1D"=w363:cluster{dbl[], dbl[]}[], "Final Temp"=w386:i32, "Init Temp"=w384:i32, "Temp Step"=w383:i32)  [unwired: 1 out]
        n152 = Subtract(x=w386, y=w384) -> (x-y=w387:i32)
        n153 = Divide(x=w387, y=w383) -> (x/y=w388:dbl)
        n154 = Increment(x=w388) -> (x+1=w385:dbl)
        n155 = for {
          N: w385 -> [_]
          tunnel: w384 -> [w395]
          tunnel: w383 -> [w396]
          tunnel: [w393] -> w375 mode=indexing
          i -> [w397]
          n156 = Multiply(x=w396, y=w397) -> (x*y=w398:i32)
          n157 = Add(x=w395, y=w398) -> (x+y=w394:i32)
          n158 = Reciprocal(x=w394) -> (1/x=w393:dbl)
        }
        n159 = call-poly <userlib>:"Linear Fit.vi"("XY-data"=w364) -> ("slopes"=w361:dbl[])  [unwired: 4 in, 6 out]
        n160 = call-poly <userlib>:"Linear Fit.vi"("XY-data"=w363) -> ("slopes"=w362:dbl[])  [unwired: 4 in, 6 out]
        n161 = Absolute Value(x=w361) -> (abs(x)=w381:dbl[])
        n162 = Absolute Value(x=w362) -> (abs(x)=w382:dbl[])
        n163 = Natural Logarithm(1:w381) -> (0:w377:dbl[])
        n164 = Natural Logarithm(1:w382) -> (0:w376:dbl[])
        n165 = Array Subset(array=w377, index=w360, length="Temps to keep (Arrhenius fit)") -> (w373:dbl[])
        n166 = Array Subset(array=w376, index=w360, length="Temps to keep (Arrhenius fit)") -> (w372:dbl[])
        n167 = Array Subset(array=w375, index=w360, length="Temps to keep (Arrhenius fit)") -> (w371:dbl[])
        n168 = Bundle(w371, w373) -> (w379:cluster{dbl[], dbl[]})  [unwired: 1 in]
        n169 = Bundle(w371, w372) -> (w380:cluster{dbl[], dbl[]})  [unwired: 1 in]
        n170 = Build Array(w379, w380) -> (w368:cluster{dbl[], dbl[]}[])
        n171 = call-poly <userlib>:"Linear Fit.vi"("XY-data"=w368) -> ("Best Fits"=w367:cluster{"X-array":dbl[], "Y-array":dbl[]}[], "XY-data out"=w366:cluster{"X-array":dbl[], "Y-array":dbl[]}[], "slopes"=w365:dbl[])  [unwired: 4 in, 4 out]
        n172 = Multiply(x=w365, y=8.617333e-05) -> (x*y=→"E_a":dbl[])
        n173 = Interleave 1D Arrays(w366, w367) -> (→"Arrhenius":cluster{"X-array":dbl[], "Y-array":dbl[]}[])
        n174 = call <vilib>:"Add State(s) to Queue__jki_lib_state_machine.vi"("State(s) in (\"\")"=w392) -> ("States Out"=w391:string)  [unwired: 14 in]
      }
      frame "Analysis: Lifespan" {
        w403 = 3600
        # "Template Separator\n(You can make a copy of, or modify, this frame)"
        n175 = Unbundle By Name(w416) -> ("G2T 1D"=w427:cluster{dbl[], dbl[]}[], "G4T 1D"=w426:cluster{dbl[], dbl[]}[], "Final Temp"=w423:i32, "Init Temp"=w415:i32, "Temp Step"=w414:i32)  [unwired: 3 out]
        n176 = Subtract(x=w423, y=w415) -> (x-y=w424:i32)
        n177 = Divide(x=w424, y=w414) -> (x/y=w425:dbl)
        n178 = Increment(x=w425) -> (x+1=w413:dbl)
        n179 = for {
          N: w413 -> [_]
          tunnel: w415 -> [w439]
          tunnel: w414 -> [w438]
          tunnel: [w437] -> w412 mode=indexing
          i -> [w440]
          n180 = Multiply(x=w438, y=w440) -> (x*y=w441:i32)
          n181 = Add(x=w439, y=w441) -> (x+y=w437:i32)
        }
        n182 = call <userlib>:"Linear Fit (multiple).vi"("XY-data"=w427) -> ("XY-data out"=w409:cluster{"X-array":dbl[], "Y-array":dbl[]}[], "slopes"=w411:dbl[])  [unwired: 4 in, 5 out]
        n183 = call <userlib>:"Linear Fit (multiple).vi"("XY-data"=w426) -> ("XY-data out"=w408:cluster{"X-array":dbl[], "Y-array":dbl[]}[], "slopes"=w410:dbl[])  [unwired: 4 in, 5 out]
        n184 = for {
          tunnel: w409 -> [w435] mode=indexing
          tunnel: w408 -> [w436] mode=indexing
          tunnel: [w432] -> w407 mode=indexing
          tunnel: [w431] -> w406 mode=indexing
          n185 = Unbundle(w435) -> ("Y-array"=w433:dbl[])  [unwired: 1 out]
          n186 = Unbundle(w436) -> ("Y-array"=w434:dbl[])  [unwired: 1 out]
          n187 = call-poly <vilib>:"Mean.vi"("X"=w434) -> ("mean"=w431:dbl)  [unwired: 1 out]
          n188 = call-poly <vilib>:"Mean.vi"("X"=w433) -> ("mean"=w432:dbl)  [unwired: 1 out]
        }
        n189 = Divide(x=w407, y=w411) -> (x/y=w405:dbl[])
        n190 = Divide(x=w406, y=w410) -> (x/y=w404:dbl[])
        n191 = Divide(x=w405, y=w403) -> (x/y=w401:dbl[])
        n192 = Divide(x=w404, y=w403) -> (x/y=w402:dbl[])
        n193 = Array Subset(array=w401, length="Temps to keep (Lifespan)") -> (w419:dbl[])  [unwired: 1 in]
        n194 = Array Subset(array=w402, length="Temps to keep (Lifespan)") -> (w418:dbl[])  [unwired: 1 in]
        n195 = Array Subset(array=w412, length="Temps to keep (Lifespan)") -> (w417:i32[])  [unwired: 1 in]
        n196 = Absolute Value(x=w419) -> (abs(x)=w399:dbl[])
        n197 = Absolute Value(x=w418) -> (abs(x)=w400:dbl[])
        n198 = Bundle(w417, w399) -> (w421:cluster{i32[], dbl[]})  [unwired: 1 in]
        n199 = Bundle(w417, w400) -> (w422:cluster{i32[], dbl[]})  [unwired: 1 in]
        n200 = Build Array(w421, w422) -> ()  [unwired: 1 out]
        n201 = call <vilib>:"Add State(s) to Queue__jki_lib_state_machine.vi"("State(s) in (\"\")"=w430) -> ("States Out"=w429:string)  [unwired: 14 in]
      }
    }
  }
  "error out" <- w1
